vi "ParseClients.vi"(0 "Text in":string, 1 "HTML in":string) -> (2 "Text out":string, 3 "success?":bool, 4 "HTML out":string)   [LabVIEW 2016]
doc: "Parses HTML and color codes clients"
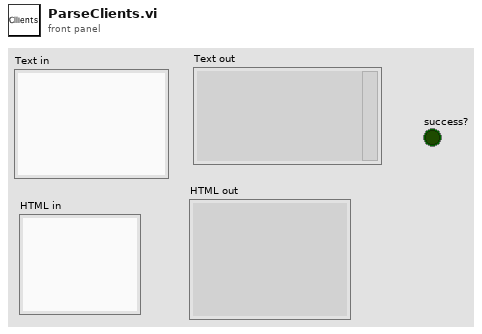
[diagram p1: front panel]
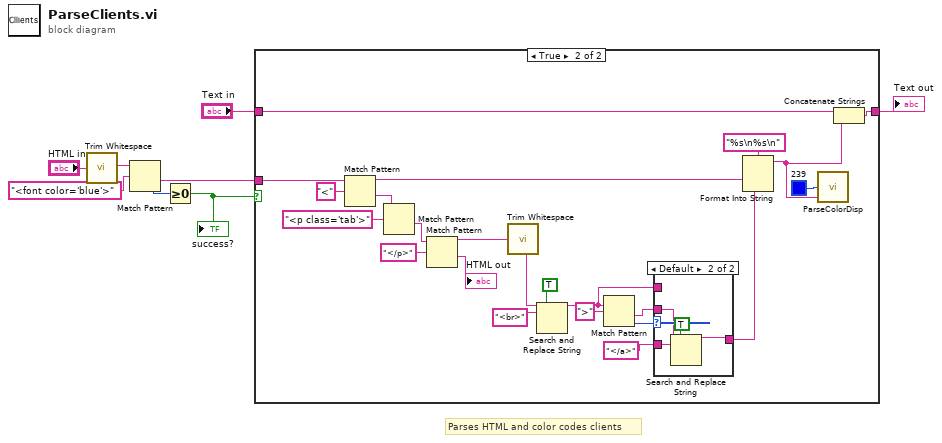
[diagram p0: block diagram]
diagram:
  # "Parses HTML and color codes clients"
  n1 = call <vilib>:"Trim Whitespace.vi"("string"="HTML in") -> ("trimmed string"=w4:string)  [unwired: 1 in]
  n2 = Match Pattern(string=w4, regular expression="<font color='blue'>") -> (after substring=w8:string, offset past match=w5:i32)  [unwired: 1 in, 2 out]
  n3 = Greater Or Equal To 0?(x=w5) -> (x >= 0?=w1:bool)
  "success?" <- w1
  n4 = case shown="True" w1 {
    tunnel: w8 -> [_ w14]
    tunnel: "Text in" -> [w9 w12]
    tunnel: [w9 w11] -> w2
    frame False {
    }
    frame True {
      n5 = Match Pattern(string=w14, regular expression="<") -> (before substring=w21:string, after substring=w17:string)  [unwired: 1 in, 2 out]
      n6 = Match Pattern(string=w17, regular expression="<p class='tab'>") -> (after substring=w19:string)  [unwired: 1 in, 3 out]
      n7 = Match Pattern(string=w19, regular expression="</p>") -> (before substring=w22:string, after substring=→"HTML out":string)  [unwired: 1 in, 2 out]
      n8 = call <vilib>:"Trim Whitespace.vi"("string"=w22) -> ("trimmed string"=w26:string)  [unwired: 1 in]
      n9 = Search and Replace String(replace all?=TRUE ("replace all? (F)"), input string=w26, search string="<br>") -> (result string=w32:string)  [unwired: 5 in, 3 out]
      n10 = Match Pattern(string=w32, regular expression=">") -> (after substring=w29:string, offset past match=w31:i32)  [unwired: 1 in, 2 out]
      n11 = case shown="Default" w31 {
        tunnel: "</a>" ("search string") -> [_ w36]
        tunnel: w29 -> [_ w35]
        tunnel: [w33 w34] -> w30
        tunnel: w32 -> [w33 _]
        frame -1 {
        }
        frame Default {
          n12 = Search and Replace String(replace all?=TRUE ("replace all? (F)"), input string=w35, search string=w36) -> (result string=w34:string)  [unwired: 5 in, 3 out]
        }
      }
      n13 = Format Into String(format string="%s\n%s\n" ("regular expression"), w21, w30) -> (resulting string=w10:string)  [unwired: 2 in, 1 out]
      n14 = call "ParseColorDisp.vi"("text"=w10, "text color(black)"=u32 239) -> ()  [unwired: 2 in, 1 out]
      n15 = Concatenate Strings(w12, w10) -> (w11:string)
    }
  }
  "Text out" <- w2
